vi "Configure Average.vi"(7 "Average On":bool, 8 "error in (no error)":errorcluster, 10 "Number of Averages":i32, 11 "VNA-Keysight PNA in":refnum<class "VNA-Keysight PNA.lvclass">) -> (0 "error out":errorcluster, 3 "VNA-Keysight PNA out":refnum<class "VNA-Keysight PNA.lvclass">)   [LabVIEW 2020, in "VNA-Keysight PNA.lvclass"]
doc: "Configures the average to use for the sweep"
uses:
  VNA-Keysight PNA.lvclass
  C:/Sandbox/RF Bench/Source Code/WiSpry Test Framework/Instruments/Instrument.lvclass
  Instrument.lvclass/Instrument.ctl
  Instrument.lvclass
  <instrlib>/Keysight PNA Series/Keysight PNA Series.lvlib
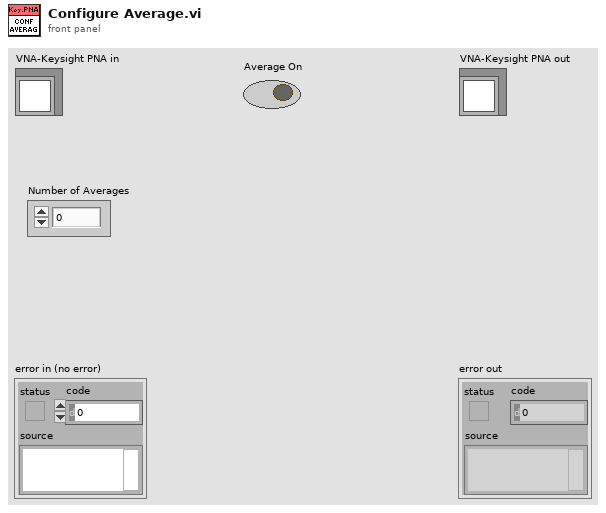
[diagram p1: front panel]
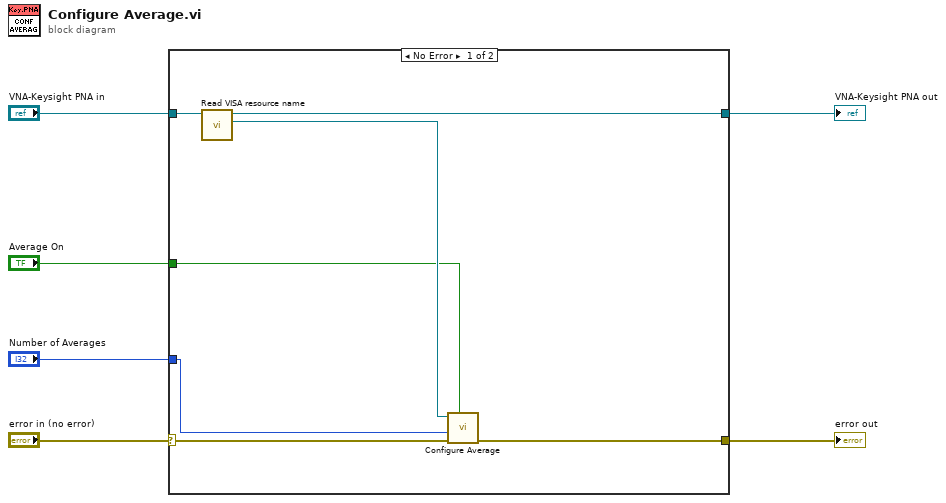
[diagram p0: block diagram]
diagram:
  n1 = case shown="No Error" "error in (no error)" {
    selector: "error in (no error)" -> [w11 w14]
    tunnel: [w12 w15] -> w1
    tunnel: "VNA-Keysight PNA in" -> [w13 w15]
    tunnel: [w9 w14] -> w2
    tunnel: "Number of Averages" -> [w10 _]
    tunnel: "Average On" -> [w7 _]
    frame No Error {
      n2 = call "Read VISA resource name.vi"("Instrument in"=w13) -> ("VISA resource name"=w8:refnum<visa-resource-name>, "Instrument out"=w12:refnum<class "VNA-Keysight PNA.lvclass">)  [unwired: 9 in]
      n3 = call <instrlib>:"Configure Average.vi"("Enable Average (F: Disable)"=w7, "error in (no error)"=w11, "Average Count (1)"=w10, "VISA resource name"=w8) -> ("error out"=w9:errorcluster)  [unwired: 6 in, 1 out]
    }
    frame Error {
    }
  }
  "error out" <- w2
  "VNA-Keysight PNA out" <- w1
